vi "PXI-Dequeue AO.vi"(0 "AO Tasks":T1[](array[typedef])=[{"Task name"="AO02", "Task"="", "Dual-channel task?"=FALSE, "Regenerate?"=FALSE, "Clear?"=FALSE}], 11 "error in (no error)":errorcluster) -> (8 "AO Waveforms":dbl[][](array[numeric]), 15 "error out":errorcluster)   [LabVIEW 2015]
uses:
  Type Defs/Task Struct.ctl
panel:
  out "Waveform Graph":dbl[][](graph)
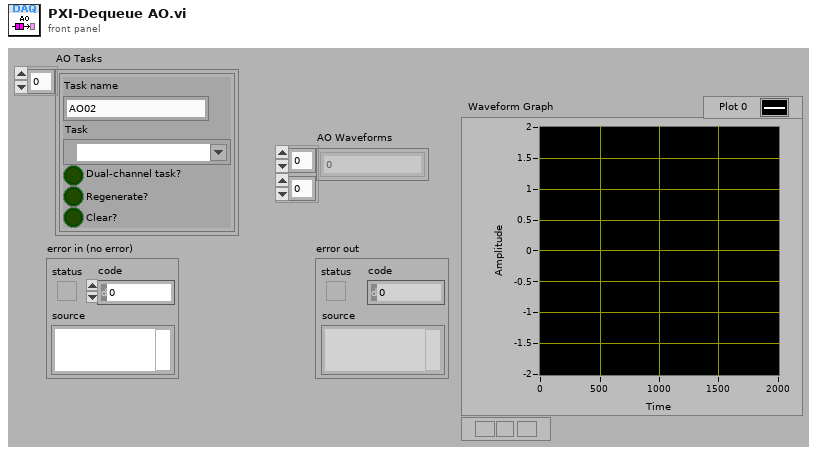
[diagram p1: front panel]
types:
  T1 = typedef "Task Struct.ctl" = cluster{"Task name":string, "Task":refnum<k21>, "Dual-channel task?":bool, "Regenerate?":bool, "Clear?":bool}
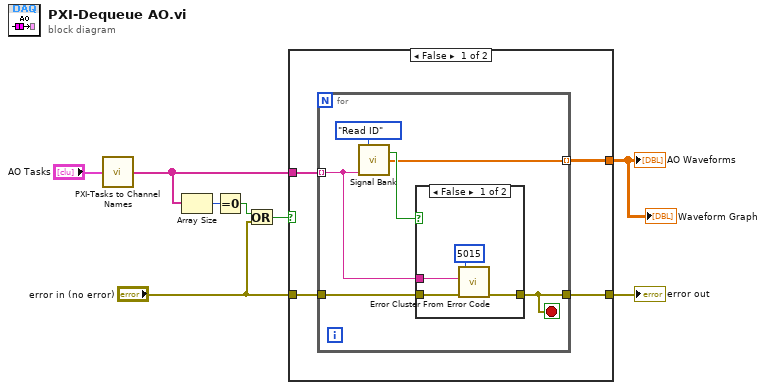
[diagram p0: block diagram]
diagram:
  n1 = call "PXI-Tasks to Channel Names.vi"("Array"="AO Tasks") -> ("Channel Names"=w2:string[])
  n2 = Array Size(array=w2) -> (size(s)=w7:i32)
  n3 = Equal To 0?(x=w7) -> (x = 0?=w5:bool)
  n4 = Or(x=w5, y="error in (no error)") -> (x .or. y?=w6:bool)
  n5 = case shown="False" w6 {
    tunnel: [w11 w24] -> w8
    tunnel: "error in (no error)" -> [w12 w24]
    tunnel: w2 -> [w9 _]
    tunnel: [w10 _] -> w4
    frame False {
      n6 = for {
        tunnel: w9 -> [w14] mode=indexing
        tunnel: [w15] -> w10 mode=indexing
        tunnel: w12 -> [w18]
        tunnel: [w13] -> w11
        stop <- w13 stop-if-true
        n7 = call "Signal Bank.vi"("Action"=enum16{"Add", "Replace ID", "Read ID", "Clear"}."Read ID", "ID"=w14) -> ("Found?"=w16:bool, "1D Data Out"=w15:dbl[])  [unwired: 12 in]
        n8 = case shown="False" w16 {
          tunnel: w18 -> [w22 w23]
          tunnel: [w21 w23] -> w13
          tunnel: w14 -> [w19 _]
          frame False {
            n9 = call <vilib>:"Error Cluster From Error Code.vi"("error in (no error)"=w22, "error message (\"\")"=w19, "error code (0)"=5015) -> ("error out"=w21:errorcluster)  [unwired: 6 in]
          }
          frame True {
          }
        }
      }
    }
    frame True {
    }
  }
  "error out" <- w8
  "AO Waveforms" <- w4
  "Waveform Graph" <- w4
